vi "Receive Link.vi"(8 "error in":errorcluster, 9 "GUI Queue In":refnum<queue>, 10 "Logger Queue In":refnum<queue>, 11 "Receive Queue In":refnum<queue>) -> (0 "error out":errorcluster)   [LabVIEW 2016]
uses:
  Message Format.ctl
  StateDef_generic.ctl
  <vilib>/addons/zeromq/socket_type.ctl
  <vilib>/addons/zeromq/socket_options.ctl
  <vilib>/addons/zeromq/zmq_context.lvclass
  <vilib>/addons/zeromq/zmq_socket.lvclass
  <vilib>/addons/zeromq/zeromq.lvlib
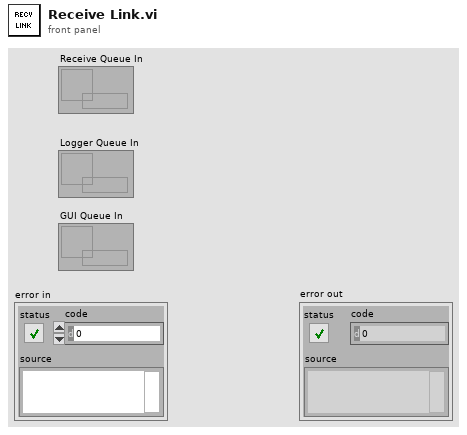
[diagram p1: front panel]
types:
  T1 = typedef "StateDef_generic.ctl" = enum16{"Initialize", "Running", "Exit"}
  T2 = typedef "zeromq.lvlib/socket_options.ctl" = enum8{"NONE", "ZMQ_HWM", "<2>", "ZMQ_SWAP", "ZMQ_AFFINITY", "ZMQ_IDENTITY", "ZMQ_SUBSCRIBE", "ZMQ_UNSUBSCRIBE", "ZMQ_RATE", "ZMQ_RECOVERY_IVL", "ZMQ_MCAST_LOOP", "ZMQ_SNDBUF", "ZMQ_RCVBUF", "ZMQ_RCVMORE", "ZMQ_FD", "ZMQ_EVENTS", "ZMQ_TYPE", "ZMQ_LINGER", "ZMQ_RECONNECT_IVL", "ZMQ_BACKLOG", "ZMQ_RECOVERY_IVL_MSEC", "ZMQ_RECONNECT_IVL_MAX", "ZMQ_MAXMSGSIZE", "ZMQ_SNDHWM", "ZMQ_RCVHWM", "ZMQ_MULTICAST_HOPS", "<26>", "ZMQ_RCVTIMEO", "ZMQ_SNDTIMEO", "<29>", "<30>", "ZMQ_IPV4ONLY", "ZMQ_LAST_ENDPOINT", "ZMQ_ROUTER_MANDATORY", "ZMQ_TCP_KEEPALIVE", "ZMQ_TCP_KEEPALIVE_CNT", "ZMQ_TCP_KEEPALIVE_IDLE", "ZMQ_TCP_KEEPALIVE_INTVL", "ZMQ_TCP_ACCEPT_FILTER", "ZMQ_DELAY_ATTACH_ON_CONNECT", "ZMQ_XPUB_VERBOSE"}
  T3 = typedef "zeromq.lvlib/socket_type.ctl" = enum8{"ZMQ_PAIR", "ZMQ_PUB", "ZMQ_SUB", "ZMQ_REQ", "ZMQ_REP", "ZMQ_DEALER", "ZMQ_ROUTER", "ZMQ_PULL", "ZMQ_PUSH", "ZMQ_XPUB", "ZMQ_XSUB"}
  T4 = typedef "Message Format.ctl" = cluster{"header":string, "data":variant}
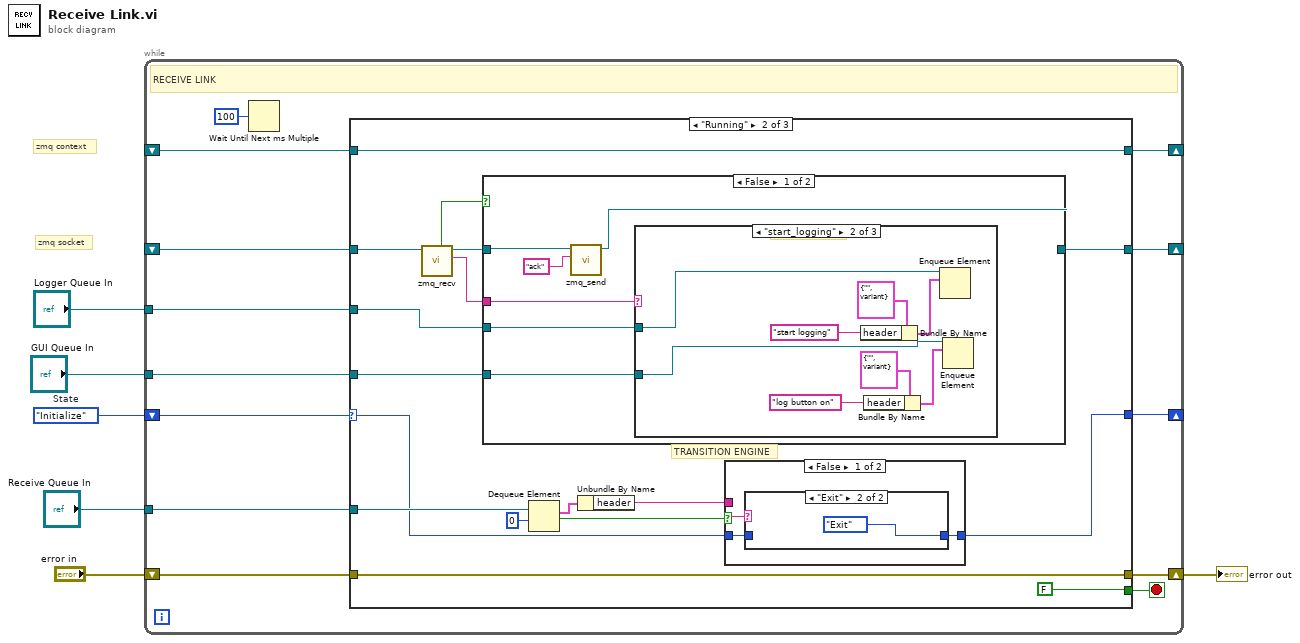
[diagram p0: block diagram]
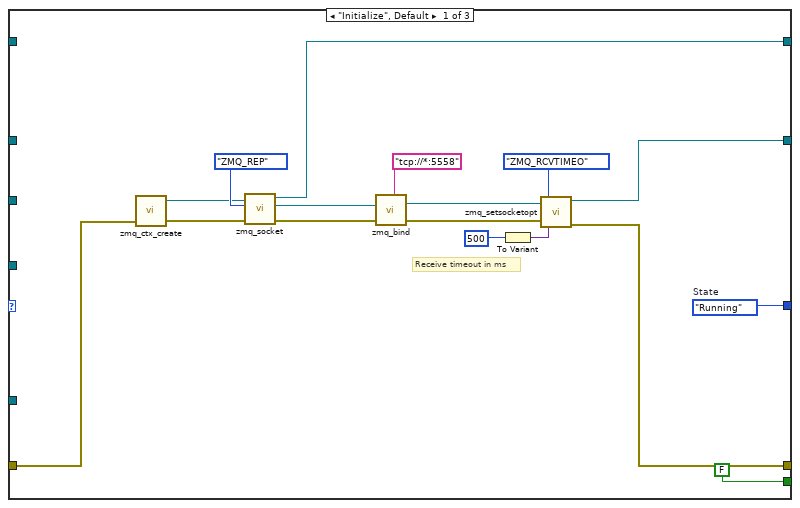
[diagram p2: hidden frame]
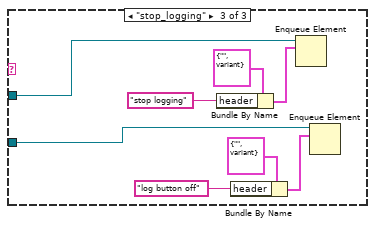
[diagram p6: hidden frame]
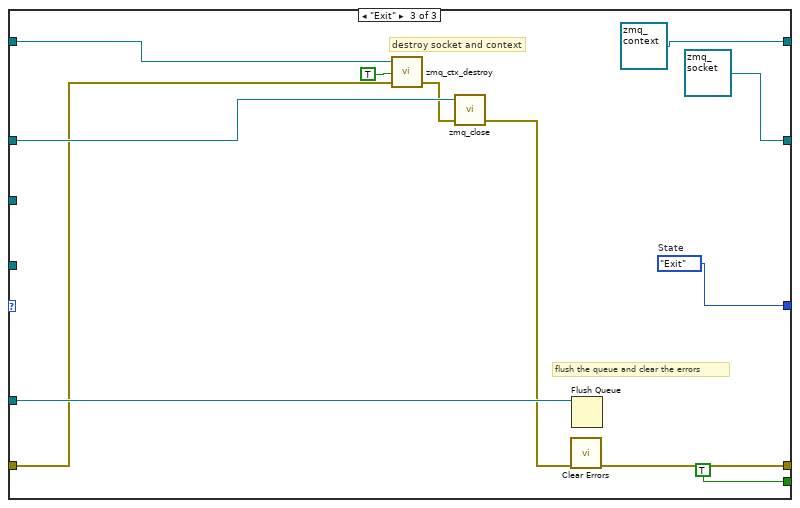
[diagram p8: hidden frame]
diagram:
  w4 = StateDef_generic."Initialize"  # State
  # "zmq socket"
  # "zmq context"
  n1 = while {
    shift-right: [w19] -> w3
    shift-left: "error in" -> [w12]
    shift-right: [w17] -> _
    shift-left: _ -> [w16]
    shift-right: [w15] -> _
    shift-left: _ -> [w14]
    tunnel: "Receive Queue In" -> [w11]
    shift-right: [w8] -> _
    shift-left: w4 -> [w13]
    tunnel: "Logger Queue In" -> [w9]
    tunnel: "GUI Queue In" -> [w7]
    stop <- w10 stop-if-true
    # "RECEIVE LINK"
    n2 = Wait Until Next ms Multiple(millisecond multiple=u32 100) -> ()  [unwired: 1 out]
    n3 = case shown="\"Running\"" w13 {
      selector: w13 -> [_ w46 _]
      tunnel: [w36 w47 w83] -> w19
      tunnel: [w35 w49 refnum<class "zmq_socket.lvclass"> refnum ("socket out")] -> w17
      tunnel: w16 -> [_ w44 w91]
      tunnel: [w24 w53 refnum<class "zmq_context.lvclass"> refnum ("context out")] -> w15
      tunnel: w14 -> [_ w53 w94]
      tunnel: w12 -> [w25 w47 w85]
      tunnel: [w21 w39 w92] -> w8
      tunnel: w11 -> [_ w50 w88]
      tunnel: [FALSE FALSE TRUE] -> w10
      tunnel: w9 -> [_ w40 _]
      tunnel: w7 -> [_ w37 _]
      frame "Initialize", Default {
        w21 = StateDef_generic."Running"  # State
        # "Receive timeout in ms"
        n4 = call <vilib>:"zmq_ctx_create.vi"("error in"=w25) -> ("error out"=w29:errorcluster, "context out"=w26:refnum<class "zmq_context.lvclass">)  [unwired: 3 in]
        n5 = call <vilib>:"zmq_socket.vi"("error in"=w29, "socket type"=socket_type."ZMQ_REP", "context in"=w26) -> ("error out"=w22:errorcluster, "socket out"=w27:refnum<class "zmq_socket.lvclass">, "context out"=w24:refnum<class "zmq_context.lvclass">)  [unwired: 2 in]
        n6 = call <vilib>:"zmq_bind.vi"("error in"=w22, "endpoint"="tcp://*:5558", "socket in"=w27) -> ("error out"=w31:errorcluster, "socket out"=w23:refnum<class "zmq_socket.lvclass">)  [unwired: 1 in]
        n7 = To Variant(anything=500) -> (Variant=w34:variant)
        n8 = call <vilib>:"zmq_setsocketopt.vi"("error in"=w31, "value"=w34, "option"=socket_options."ZMQ_RCVTIMEO", "socket in"=w23) -> ("error out"=w36:errorcluster, "socket out"=w35:refnum<class "zmq_socket.lvclass">)  [unwired: 2 in]
      }
      frame "Running" {
        # "TRANSITION ENGINE"
        n9 = call <vilib>:"zmq_recv.vi"("socket in"=w44) -> ("data"=w41:string, "socket out"=w43:refnum<class "zmq_socket.lvclass">, "timeout?"=w42:bool)  [unwired: 4 in, 2 out]
        n10 = case shown="False" w42 {
          tunnel: w43 -> [w63 w82]
          tunnel: [w61 w82] -> w49
          tunnel: w41 -> [w65 _]
          tunnel: w40 -> [w62 _]
          tunnel: w37 -> [w60 _]
          frame False {
            # "parse message"
            n11 = call <vilib>:"zmq_send.vi"("data"="ack", "socket in"=w63) -> ("socket out"=w61:refnum<class "zmq_socket.lvclass">)  [unwired: 5 in, 1 out]
            n12 = case shown="\"start_logging\"" w65 {
              tunnel: w62 -> [_ w70 w78]
              tunnel: w60 -> [_ w66 w74]
              frame "other", Default {
              }
              frame "start_logging" {
                n13 = Bundle By Name(cluster=T4 {"header"="", "data"=variant} ("msg format"), "header"="start logging") -> (w71:T4)
                n14 = Bundle By Name(cluster=T4 {"header"="", "data"=variant} ("msg format"), "header"="log button on") -> (w67:T4)
                n15 = Enqueue Element(queue=w70, element=w71) -> ()  [unwired: 2 in, 3 out]
                n16 = Enqueue Element(queue=w66, element=w67) -> ()  [unwired: 2 in, 3 out]
              }
              frame "stop_logging" {
                n17 = Bundle By Name(cluster=T4 {"header"="", "data"=variant} ("msg format"), "header"="stop logging") -> (w79:T4)
                n18 = Bundle By Name(cluster=T4 {"header"="", "data"=variant} ("msg format"), "header"="log button off") -> (w75:T4)
                n19 = Enqueue Element(queue=w78, element=w79) -> ()  [unwired: 2 in, 3 out]
                n20 = Enqueue Element(queue=w74, element=w75) -> ()  [unwired: 2 in, 3 out]
              }
            }
          }
          frame True {
          }
        }
        n21 = Dequeue Element(queue=w50, timeout in ms (-1)=0) -> (element=w51:T4, timed out?=w38:bool)  [unwired: 1 in, 2 out]
        n22 = Unbundle By Name(w51) -> ("header"=w45:string)
        n23 = case shown="False" w38 {
          tunnel: w45 -> [w54 _]
          tunnel: [w56 w59] -> w39
          tunnel: w46 -> [w55 w59]
          frame False {
            n24 = case shown="\"Exit\"" w54 {
              tunnel: [w57 StateDef_generic."Exit" ("State")] -> w56
              tunnel: w55 -> [w57 _]
              frame "any other", Default {
              }
              frame "Exit" {
              }
            }
          }
          frame True {
          }
        }
      }
      frame "Exit" {
        w92 = StateDef_generic."Exit"  # State
        # "flush the queue and clear the errors"
        # "destroy socket and context"
        n25 = call <vilib>:"zmq_ctx_destroy.vi"("error in"=w85, "reap? (F)"=TRUE, "context in"=w94) -> ("error out"=w86:errorcluster)  [unwired: 2 in]
        n26 = call <vilib>:"zmq_close.vi"("error in"=w86, "socket"=w91) -> ("error out"=w84:errorcluster)  [unwired: 3 in]
        n27 = call <vilib>:"Clear Errors.vi"("error in (no error)"=w84) -> ("error out"=w83:errorcluster)  [unwired: 5 in, 1 out]
        n28 = Flush Queue(queue=w88) -> ()  [unwired: 1 in, 3 out]
      }
    }
  }
  "error out" <- w3
